vi "Periodic Tasks.vi"(8 "error in":errorcluster) -> ()   [LabVIEW 2016]
doc: "This VI runs in parallel to other tasks. It can contain as many user-defined periodic loops as you need. These can carry out PID or other sorts of timed response."
uses:
  <vilib>/Rock Robotics/WPI/Accelerometer/WPI_AccelerometerRange.ctl
  <vilib>/Rock Robotics/WPI/DriverStation/WPI_DriverStationRobotMode2.ctl
  <vilib>/Rock Robotics/WPI/Utilities/WPI_GetSetVariantRefNum.vi
  Robot Global Data.vi
  <vilib>/Rock Robotics/WPI/RobotDrive/WPI_RobotDriveArcadeDrive_Standard(NoSaturation).vi
  <vilib>/Rock Robotics/Network Tables/NT Write Numeric Array.vi
  <vilib>/Rock Robotics/Network Tables/NT Read Boolean.vi
  <vilib>/Rock Robotics/Network Tables/NT Write Boolean Array.vi
  <vilib>/Rock Robotics/WPI/Accelerometer/InternalAccelerometer/WPI_AccelerometerInternalOpen.vi
panel:
  in  "Drive Straight on Button":i32=99
  out "Joy Y":dbl
  in  "Accel Range":T1
  out "X Acceleration":dbl
  out "Y Acceleration":dbl
  out "Z Acceleration":dbl
  out "Joy X":dbl
  out "Angle":dbl
  # "Joy 0 Control"
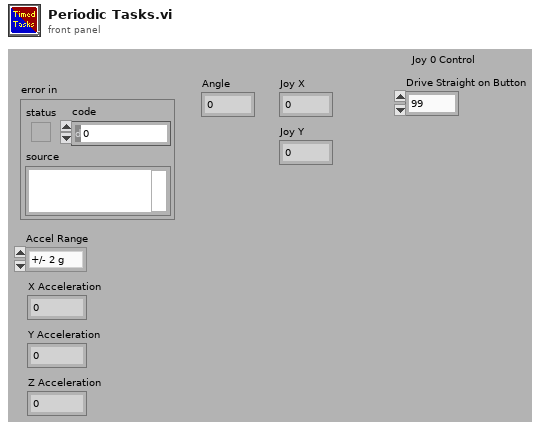
[diagram p1: front panel]
types:
  T1 = typedef "WPI_AccelerometerRange.ctl" = enum16{"+/- 2 g", "+/- 4 g", "+/- 8 g"}
  T2 = typedef "WPI_GyroDevRef.ctl" = cluster{"DevStatus":errorcluster, "Analog Channel":T3, "Offset":dbl, "Gain (VoltsPerDegree/Second)":dbl, "Gyro Type":enum16{"Analog", "XRS450"}, "Handle":i32, "SPI Bus":T4, "Device Found":bool, "Sample Rate":dbl, "Calibrate On Open":bool}
  T3 = typedef "FPGA_AIChannel.ctl" = enum8{"AI 0", "AI 1", "AI 2", "AI 3", "AI MXP 0", "AI MXP 1", "AI MXP 2", "AI MXP 3", "Invalid"}
  T4 = typedef "spi_bus.ctl" = enum16{"SPI On-Board, CS0", "SPI On-Board, CS1", "SPI On-Board, CS2", "SPI On-Board, CS3", "SPI MXP", "Invalid"}
  T5 = typedef "WPI_AccelerometerDevRef.ctl" = cluster{"DevStatus":errorcluster, "Scaling":T6, "Analog Channels":T7, "I2C Bus":T8, "SPI Bus":T4, "Accel Range":T9, "ADXL Axes":T10, "Handle":i32, "Device Address":u8, "Accel Type":enum16{"Analog", "ADXL345 I2C", "ADXL345 SPI", "Internal", "ADXL362 SPI"}}
  T6 = typedef "WPI_AccelerometerScaling.ctl" = cluster{"Gain (VoltsPerG)":dbl, "Center Voltage":dbl}
  T7 = typedef "WPI_AccelerometerAnalogChannels.ctl" = cluster{"X-Axis":T3, "Y-Axis":T3, "Z-Axis":T3}
  T8 = typedef "i2c_bus.ctl" = enum16{"I2C On-Board", "I2C MXP", "Invalid"}
  T9 = typedef "ADXL345 Range.ctl" = u8
  T10 = typedef "WPI_AccelerometerADXL345 Axes.ctl" = cluster{"X-Axis":bool, "Y-Axis":bool, "Z-Axis":bool}
  T11 = typedef "WPI_JoystickDevRef.ctl" = cluster{"Device":T12}
  T12 = typedef "WPI_JoystickDeviceEnum.ctl" = enum16{"USB 0", "USB 1", "USB 2", "USB 3", "USB 4", "USB 5"}
  T13 = typedef "WPI_RobotDriveDevRef.ctl" = cluster{"DevStatus":errorcluster, "Motors[]":T14[], "Square Inputs":bool, "Max Output":dbl}
  T14 = typedef "WPI_MotorControlDeviceRef.ctl" = cluster{"DeviceStatus":errorcluster, "Type":T15, "PWM":cluster{"PWM Channel":T16, "DeadBand":T17}, "CAN":cluster{"Device Number":u8, "SetOutput VI Ref":variant, "GetOutput VI Ref":variant, "Enable VI Ref":variant, "Disable VI Ref":variant, "Data":variant}, "Invert":bool}
  T15 = typedef "WPI_MotorControlType.ctl" = enum16{"PWM", "CAN"}
  T16 = typedef "FPGA_DIOPWMChannel.ctl" = enum8{"PWM 0", "PWM 1", "PWM 2", "PWM 3", "PWM 4", "PWM 5", "PWM 6", "PWM 7", "PWM 8", "PWM 9", "PWM MXP 0", "PWM MXP 1", "PWM MXP 2", "PWM MXP 3", "PWM MXP 4", "PWM MXP 5", "PWM MXP 6", "PWM MXP 7", "PWM MXP 8", "PWM MXP 9", "Invalid"}
  T17 = typedef "WPI_PWMDeadband.ctl" = cluster{"Name":string, "maxPositivePwm":i32, "minPositivePwm":i32, "centerPwm":i32, "maxNegativePwm":i32, "minNegativePwm":i32, "angularRange":u16}
  T18 = cluster{"JoystickDevRef":T11, "RobotDriveDevRef":T13}
  T19 = cluster{"X-Axis":dbl, "Y-Axis":dbl, "Z-Axis":dbl}
  T20 = typedef "WPI_DriverStationRobotMode2.ctl" = enum16{"Autonomous Disabled", "Autonomous Enabled", "Teleop Disabled", "Teleop Enabled", "Disconnected", "Finish", "Test Disabled", "Test Enabled", "Emergency Stopped"}
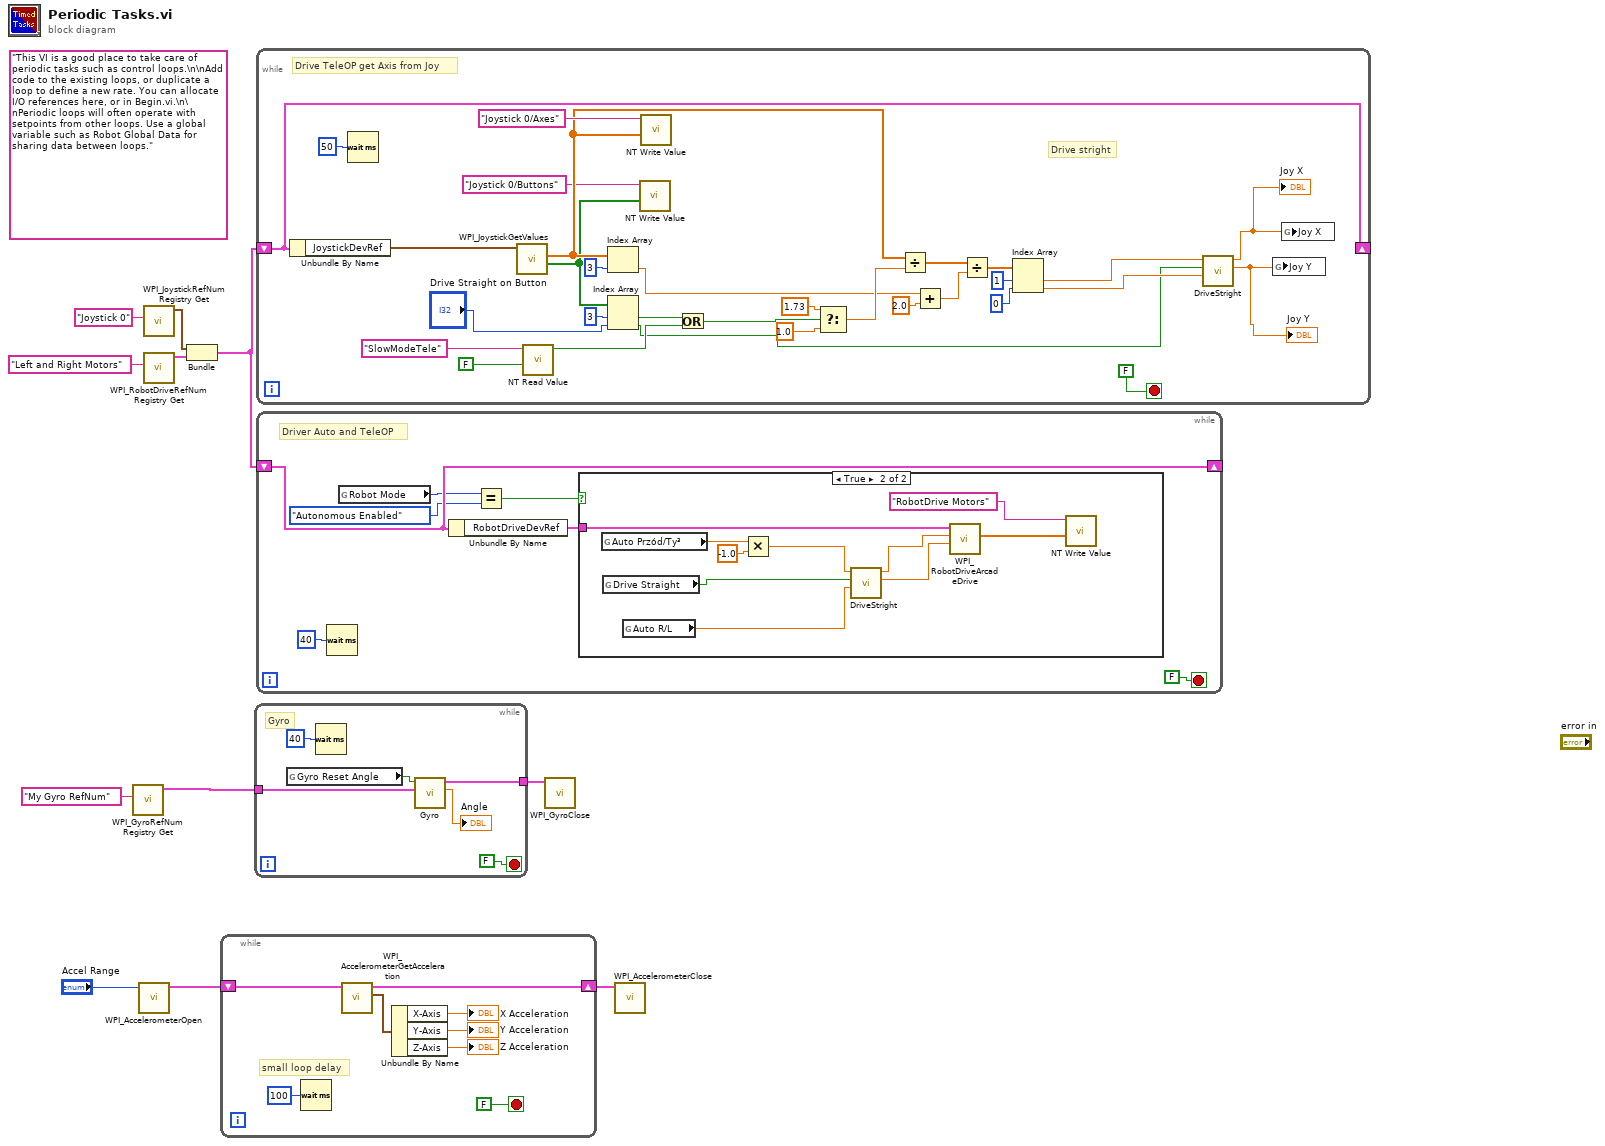
[diagram p0: block diagram]
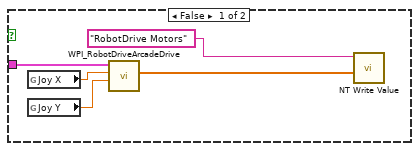
[diagram p2: hidden frame]
diagram:
  (unwired) "This VI is a good place to take care of periodic tasks such as control loops.\n\nAdd code to the existing loops, or duplicate a loop to define a new rate. You can allocate I/O references here, or in Begin.vi.\n\nPeriodic loops will often operate with setpoints from other loops. Use a global variable such as Robot Global Data for sharing data between loops."
  n1 = call <vilib>:"WPI_GyroRefNum Registry Get.vi"("refnum name"="My Gyro RefNum") -> ("GyroDevRef"=w5:T2)  [unwired: 9 in, 1 out]
  n2 = call-poly <vilib>:"WPI_AccelerometerOpen.vi"("Accel Range"="Accel Range") -> ("AccelerometerDevRef"=w3:T5)  [unwired: 9 in, 1 out]
  n3 = call <vilib>:"WPI_JoystickRefNum Registry Get.vi"("refnum name"="Joystick 0") -> ("JoystickDevRef"=w9:T11)  [unwired: 1 in, 9 out]
  n4 = call <vilib>:"WPI_RobotDriveRefNum Registry Get.vi"("refnum name"="Left and Right Motors") -> ("RobotDriveDevRef"=w8:T13)  [unwired: 1 in, 9 out]
  n5 = Bundle("JoystickDevRef"=w9, "RobotDriveDevRef"=w8) -> (w7:T18)  [unwired: 1 out]
  n6 = while {
    shift-right: [w17] -> w2
    shift-left: w3 -> [w16]
    stop <- FALSE stop-if-true
    # "small loop delay"
    n7 = Wait (ms)(milliseconds to wait=u32 100) -> ()  [unwired: 1 out]
    n8 = call <vilib>:"WPI_AccelerometerGetAcceleration.vi"("AccelerometerDevRef"=w16) -> ("Accelerations"=w18:T19, "AccelerometerDevRef"=w17:T5)  [unwired: 8 in, 1 out]
    n9 = Unbundle By Name(w18) -> ("X-Axis"=→"X Acceleration":dbl, "Y-Axis"=→"Y Acceleration":dbl, "Z-Axis"=→"Z Acceleration":dbl)
  }
  n10 = while {
    tunnel: w5 -> [w23]
    tunnel: [w21] -> w4
    stop <- FALSE stop-if-true
    # "Gyro"
    n11 = global read "Robot Global Data.vi" "Gyro Reset Angle"() -> (w22:bool)
    n12 = Wait (ms)(milliseconds to wait=u32 40) -> ()  [unwired: 1 out]
    n13 = call "Gyro.vi"("GyroDevRef in"=w23, "Gyro Reset Angle"=w22) -> ("Angle"=→"Angle":dbl, "GyroDevRef out"=w21:T2)  [unwired: 8 in]
  }
  n14 = while {
    shift-right: [w55] -> _
    shift-left: w7 -> [w55]
    stop <- FALSE stop-if-true
    # "Drive stright"
    # "Drive TeleOP get Axis from Joy"
    n15 = Unbundle By Name(w55) -> ("JoystickDevRef"=w39:T11)
    n16 = Wait (ms)(milliseconds to wait=u32 50) -> ()  [unwired: 1 out]
    n17 = call <vilib>:"WPI_JoystickGetValues.vi"("JoystickDevRef"=w39) -> ("Buttons"=w37:bool[], "Axes"=w38:dbl[])  [unwired: 6 in, 3 out]
    n18 = call-poly <vilib>:"NT Read Value.vi"("Default Value"=FALSE, "Name"="SlowModeTele") -> ("Boolean"=w48:bool)  [unwired: 8 in, 1 out]
    n19 = Index Array(array=w38, index=3) -> (element=w41:dbl)
    n20 = Index Array(array=w37, index #1=3 ("index"), index #2="Drive Straight on Button") -> (element #1=w50:bool, element #2=w26:bool)
    n21 = call-poly <vilib>:"NT Write Value.vi"("Boolean Array"=w37, "Name"="Joystick 0/Buttons") -> ()  [unwired: 9 in, 1 out]
    n22 = call-poly <vilib>:"NT Write Value.vi"("Numeric Array"=w38, "Name"="Joystick 0/Axes") -> ()  [unwired: 9 in, 1 out]
    n23 = Or(x=w50, y=w48) -> (x .or. y?=w49:bool)
    n24 = Select(t=1.73, s=w49, f=1.0) -> (s? t:f=w51:dbl)
    n25 = Divide(x=w38, y=w51) -> (x/y=w45:dbl[])
    n26 = Add(x=w41, y=2.0) -> (x+y=w44:dbl)
    n27 = Divide(x=w45, y=w44) -> (x/y=w46:dbl[])
    n28 = Index Array(array=w46, index #1=1 ("index"), index #2=0 ("index")) -> (element #1=w31:dbl, element #2=w30:dbl)
    n29 = call "DriveStright.vi"("Joy Y in"=w30, "Drive Stright"=w26, "Joy X in"=w31) -> ("Joy Y out"=w33:dbl, "Joy X out"=w32:dbl)  [unwired: 7 in]
    "Joy X" <- w32
    "Joy Y" <- w33
    n30 = global write "Robot Global Data.vi" "Joy Y"(w33) -> ()
    n31 = global write "Robot Global Data.vi" "Joy X"(w32) -> ()
  }
  n32 = while {
    shift-right: [w62] -> _
    shift-left: w7 -> [w62]
    stop <- FALSE stop-if-true
    # "Driver Auto and TeleOP"
    n33 = Wait (ms)(milliseconds to wait=u32 40) -> ()  [unwired: 1 out]
    n34 = global read "Robot Global Data.vi" "Robot Mode"() -> (w61:T20)
    n35 = Unbundle By Name(w62) -> ("RobotDriveDevRef"=w58:T13)
    n36 = Equal?(x=w61, y=WPI_DriverStationRobotMode2."Autonomous Enabled") -> (x = y?=w59:bool)
    n37 = case shown="True" w59 {
      tunnel: w58 -> [w68 w77]
      frame False {
        n38 = global read "Robot Global Data.vi" "Joy X"() -> (w66:dbl)
        n39 = global read "Robot Global Data.vi" "Joy Y"() -> (w67:dbl)
        n40 = call-poly <vilib>:"WPI_RobotDriveArcadeDrive.vi"("Y axis value"=w67, "X axis value"=w66, "RobotDriveDevRef"=w68) -> ("Motor Values"=w64:dbl[])  [unwired: 6 in, 2 out]
        n41 = call-poly <vilib>:"NT Write Value.vi"("Numeric Array"=w64, "Name"="RobotDrive Motors") -> ()  [unwired: 9 in, 1 out]
      }
      frame True {
        n42 = global read "Robot Global Data.vi" "Auto Przód/Ty³"() -> (w74:dbl)
        n43 = global read "Robot Global Data.vi" "Drive Straight"() -> (w73:bool)
        n44 = global read "Robot Global Data.vi" "Auto R/L"() -> (w70:dbl)
        n45 = Multiply(x=w74, y=-1.0) -> (x*y=w72:dbl)
        n46 = call "DriveStright.vi"("Joy Y in"=w70, "Drive Stright"=w73, "Joy X in"=w72) -> ("Joy Y out"=w69:dbl, "Joy X out"=w71:dbl)  [unwired: 7 in]
        n47 = call-poly <vilib>:"WPI_RobotDriveArcadeDrive.vi"("Y axis value"=w69, "X axis value"=w71, "RobotDriveDevRef"=w77) -> ("Motor Values"=w76:dbl[])  [unwired: 6 in, 2 out]
        n48 = call-poly <vilib>:"NT Write Value.vi"("Numeric Array"=w76, "Name"="RobotDrive Motors") -> ()  [unwired: 9 in, 1 out]
      }
    }
  }
  n49 = call <vilib>:"WPI_GyroClose.vi"("GyroDevRef"=w4) -> ()  [unwired: 10 in, 1 out]
  n50 = call <vilib>:"WPI_AccelerometerClose.vi"("AccelerometerDevRef"=w2) -> ()  [unwired: 10 in, 1 out]
